vi "Initialize Analog Module.vi"(7 "Direction":enum16{"Input", "Output"}(ring), 8 "error in (no error)":errorcluster, 9 "FXP Type":string, 10 "Channels":u8, 11 "Module in":refnum<class "Module.lvclass">) -> (0 "error out":errorcluster, 3 "Module out":refnum<class "Module.lvclass">)   [LabVIEW 2015, in "Module.lvclass"]
uses:
  Module.lvclass
  Module Configuration.ctl
  Module.lvclass/Module.ctl
  VI/Module Loop/Module Loop.lvclass
  <vilib>/Utility/Data Type/NI_Data Type.lvlib
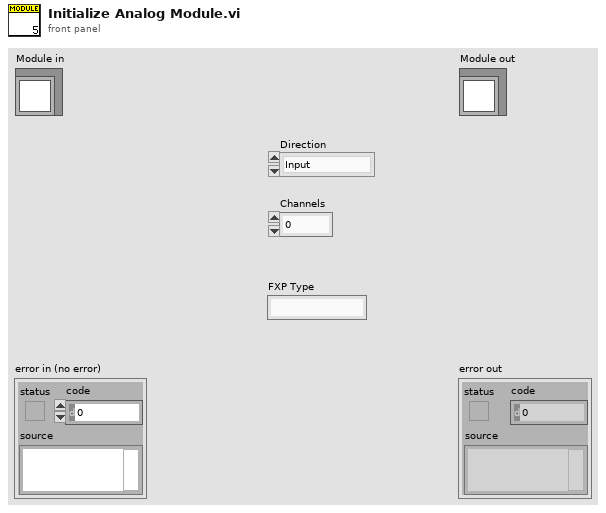
[diagram p1: front panel]
types:
  T1 = typedef "Module Loop.lvclass/Module Configuration.ctl" = cluster{"Type":string, "Direction":string, "Speed":string, "Channels":string, "FXP Type":string}
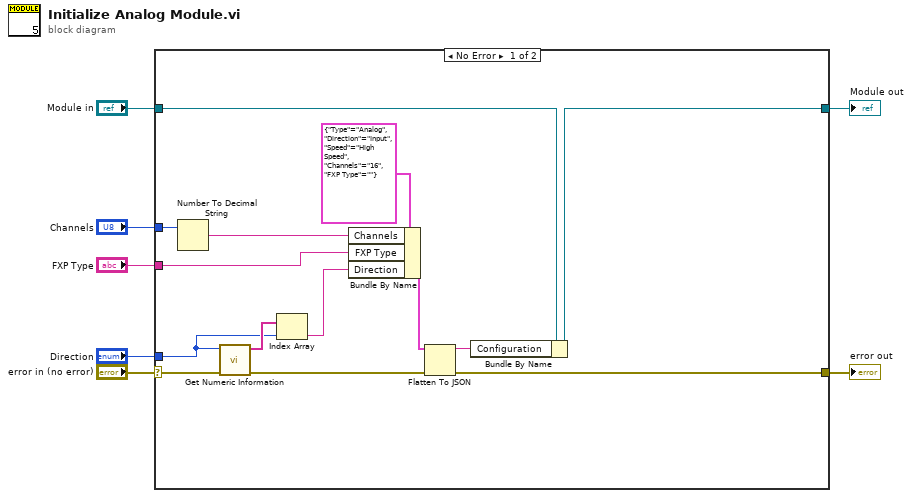
[diagram p0: block diagram]
diagram:
  n1 = case shown="No Error" "error in (no error)" {
    selector: "error in (no error)" -> [w11 w23]
    tunnel: [w17 w23] -> w6
    tunnel: [w13 w22] -> w4
    tunnel: "Module in" -> [w14 w22]
    tunnel: "Direction" -> [w8 _]
    tunnel: "Channels" -> [w20 _]
    tunnel: "FXP Type" -> [w18 _]
    frame No Error {
      n2 = Number To Decimal String(number=w20) -> (decimal integer string=w19:string)  [unwired: 1 in]
      n3 = call <vilib>:"Get Numeric Information.vi"("error in (no error)"=w11, "Variant"=w8) -> ("error out"=w10:errorcluster, "Enum Names"=w12:string[])  [unwired: 6 in, 2 out]
      n4 = Index Array(array=w12, index=w8) -> (element=w9:string)
      n5 = Bundle By Name(cluster=T1 {"Type"="Analog", "Direction"="Input", "Speed"="High Speed", "Channels"="16", "FXP Type"=""} ("Cluster"), "Channels"=w19, "FXP Type"=w18, "Direction"=w9) -> (w16:T1)
      n6 = Flatten To JSON(anything=w16, error in (no error)=w10) -> (JSON string=w15:string, 11:w17:errorcluster)  [unwired: 1 in]
      n7 = Bundle By Name(cluster=w14, "Configuration"=w15) -> (w13:refnum<class "Module.lvclass">)
    }
    frame Error {
    }
  }
  "error out" <- w6
  "Module out" <- w4
